vi "UR Client.vi"() -> ()   [LabVIEW 2016]
panel:
  out "size(s)":i32
  out "data":string
  in  "stop":bool
  in  "rcv":bool
  out "data out":string
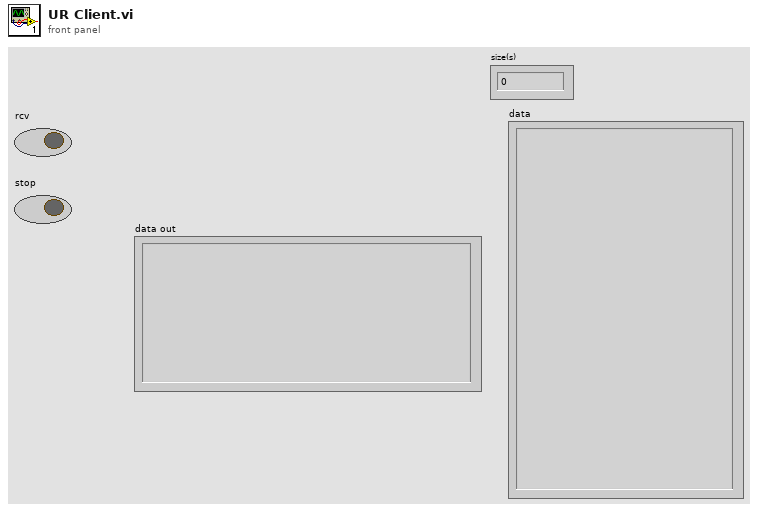
[diagram p1: front panel]
types:
  T1 = enum16{"Standard", "Buffered", "CRLF", "Immediate"}
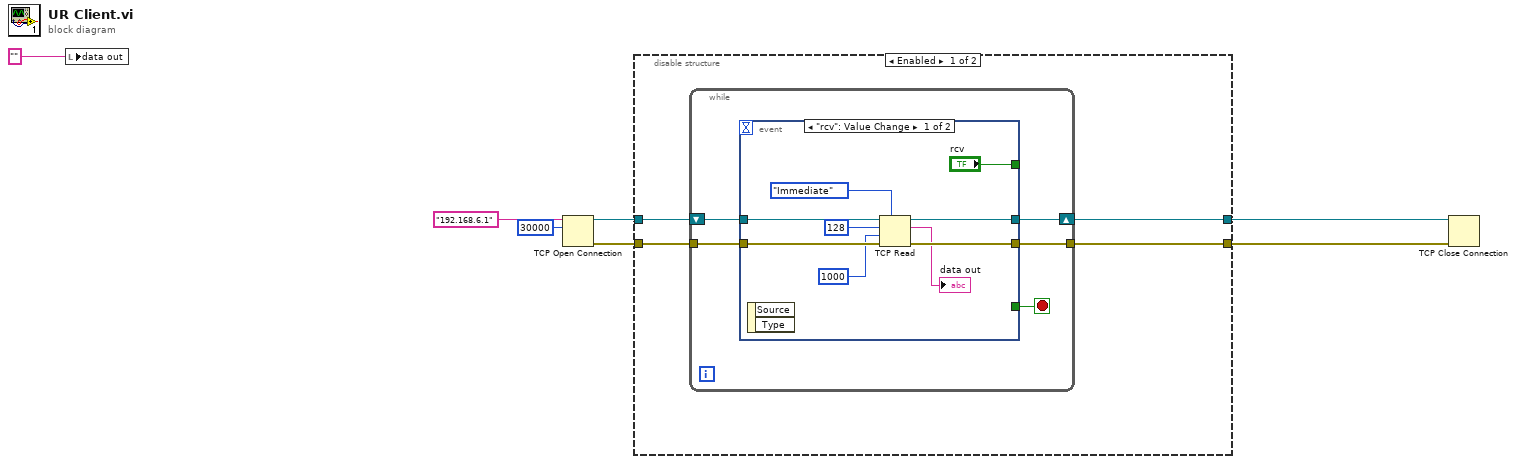
[diagram p0: block diagram]
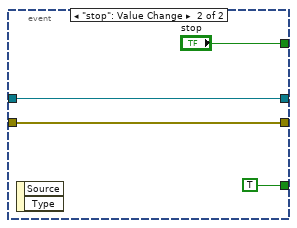
[diagram p2: hidden frame]
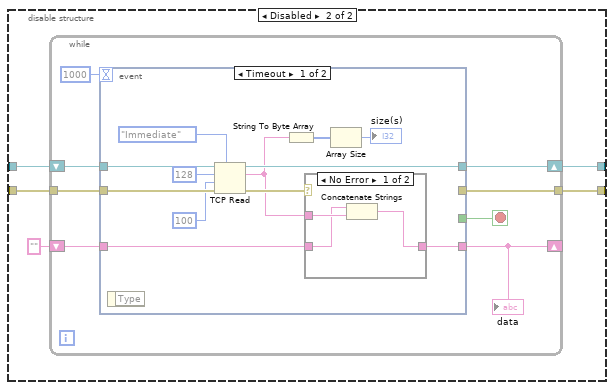
[diagram p3: hidden frame]
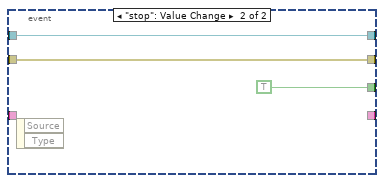
[diagram p5: hidden frame]
diagram:
  n1 = local write "data out"("" ("data out")) -> ()
  n2 = TCP Open Connection(address="192.168.6.1" ("name"), remote port or service name=u16 30000) -> (connection ID=w1:refnum<k5>, error out=w2:errorcluster)  [unwired: 3 in]
  n3 = disable-structure shown="Enabled" {
    disable-tunnel: [w11 w34] -> w7
    disable-tunnel: [w10 w33] -> w6
    disable-tunnel: w1 -> [w9 w32]
    disable-tunnel: w2 -> [w8 w31]
    frame Enabled {
      n4 = while {
        shift-right: [w16] -> w11
        shift-left: w9 -> [w13]
        tunnel: w8 -> [w14]
        tunnel: [w15] -> w10
        stop <- w12 stop-if-true
        n5 = event shown="[0] \"rcv\": Value Change" {
          selector: _ -> [_ _]
          dyn-events: _ -> [_ _]
          timeout: _ -> [_ _]
          tunnel: [w25 w28] -> w16
          tunnel: [w24 w27] -> w15
          tunnel: w14 -> [w23 w27]
          tunnel: w13 -> [w22 w28]
          tunnel: ["rcv" "stop"] -> _
          tunnel: [_ TRUE] -> w12
          event "rcv": Value Change {
            n6 = event-data() -> ()  [unwired: 1 in, 2 out]
            n7 = TCP Read(connection ID=w22, bytes to read=128, error in (no error)=w23, 7:T1."Immediate" ("mode (standard)"), 9:1000 ("timeout ms (25000)")) -> (connection ID out=w25:refnum<k5>, data out=→"data out":string, error out=w24:errorcluster)
          }
          event "stop": Value Change {
            n8 = event-data() -> ()  [unwired: 1 in, 2 out]
          }
        }
      }
    }
    frame Disabled {
      n9 = while {
        shift-right: [w42] -> w34
        shift-left: w32 -> [w39]
        tunnel: w31 -> [w40]
        tunnel: [w41] -> w33
        shift-right: [w36] -> _
        shift-left: "" -> [w35]
        stop <- w38 stop-if-true
        n10 = event shown="[0] Timeout" {
          selector: _ -> [_ _]
          dyn-events: _ -> [_ _]
          timeout: 1000 -> [_ _]
          tunnel: [w54 w61] -> w42
          tunnel: [_ w60] -> w41
          tunnel: w40 -> [w53 w60]
          tunnel: w39 -> [w52 w61]
          tunnel: [_ TRUE] -> w38
          tunnel: [w50 _] -> w36
          tunnel: w35 -> [w49 _]
          event Timeout {
            n11 = event-data() -> ()  [unwired: 1 in, 1 out]
            n12 = TCP Read(connection ID=w52, bytes to read=128, error in (no error)=w53, 7:T1."Immediate" ("mode (standard)"), 9:100 ("timeout ms (25000)")) -> (connection ID out=w54:refnum<k5>, data out=w45:string, error out=w51:errorcluster)
            n13 = String To Byte Array(string=w45) -> (unsigned byte array=w44:u8[])
            n14 = case shown="No Error" w51 {
              tunnel: w45 -> [w57 _]
              tunnel: [w56 w58] -> w50
              tunnel: w49 -> [w55 w58]
              frame No Error {
                n15 = Concatenate Strings(w55, w57) -> (w56:string)
              }
              frame Error {
              }
            }
            n16 = Array Size(array=w44) -> (size(s)=→"size(s)":i32)
          }
          event "stop": Value Change {
            n17 = event-data() -> ()  [unwired: 1 in, 2 out]
          }
        }
        "data" <- w36
      }
    }
  }
  n18 = TCP Close Connection(connection ID=w7, error in (no error)=w6) -> ()  [unwired: 1 in, 2 out]
